vi "Variant to eActor Event.vi"(8 "error in (no error)":errorcluster, 10 "Variant":variant, 11 "eActor in":refnum<class "eActor.lvclass">) -> (0 "error out":errorcluster, 2 "Event Registration Refnum":refnum<event-registration>, 3 "eActor out":refnum<class "eActor.lvclass">)   [LabVIEW 2015, in "AMS UI.lvlib" / "eActor.lvclass"]
uses:
  eActor.lvclass
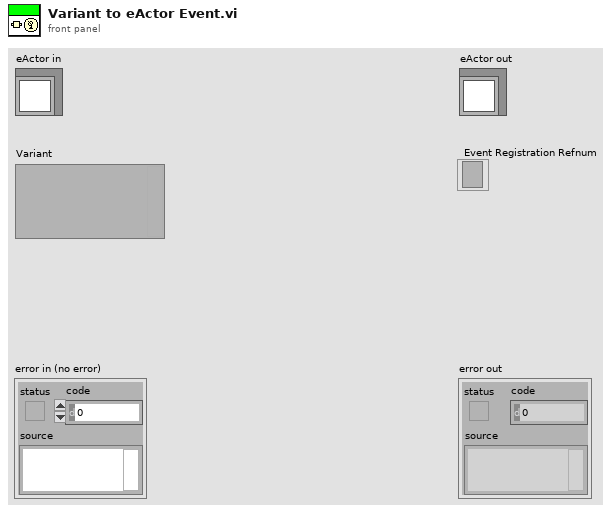
[diagram p1: front panel]
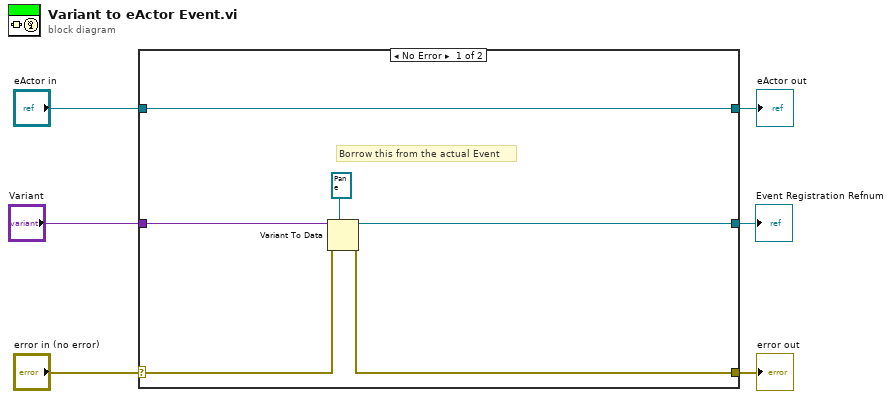
[diagram p0: block diagram]
diagram:
  n1 = case shown="No Error" "error in (no error)" {
    selector: "error in (no error)" -> [w9 w14]
    tunnel: [w8 w14] -> w5
    tunnel: [w12 w13] -> w3
    tunnel: "eActor in" -> [w12 w13]
    tunnel: "Variant" -> [w10 _]
    tunnel: [w7 _] -> w1
    frame No Error {
      # "Borrow this from the actual Event"
      n2 = Variant To Data(error in=w9, type=refnum<event-registration> refnum ("event registration refnum"), Variant=w10) -> (data=w7:refnum<event-registration>, error out=w8:errorcluster)
    }
    frame Error {
    }
  }
  "error out" <- w5
  "eActor out" <- w3
  "Event Registration Refnum" <- w1
